vi "灰度分析2.vi"() -> ()   [LabVIEW 2018]
uses:
  <vilib>/vision/NI_Vision_Development_Module.lvlib
panel:
  out "error out":errorcluster
  out "波形图 2":cluster{"x0":sgl, "dx":sgl, "Pixels Line":sgl[]}(graph)
  out "波形图":sgl[](graph)
  out "Image":T1(plugin-control)
  in  "路径":path
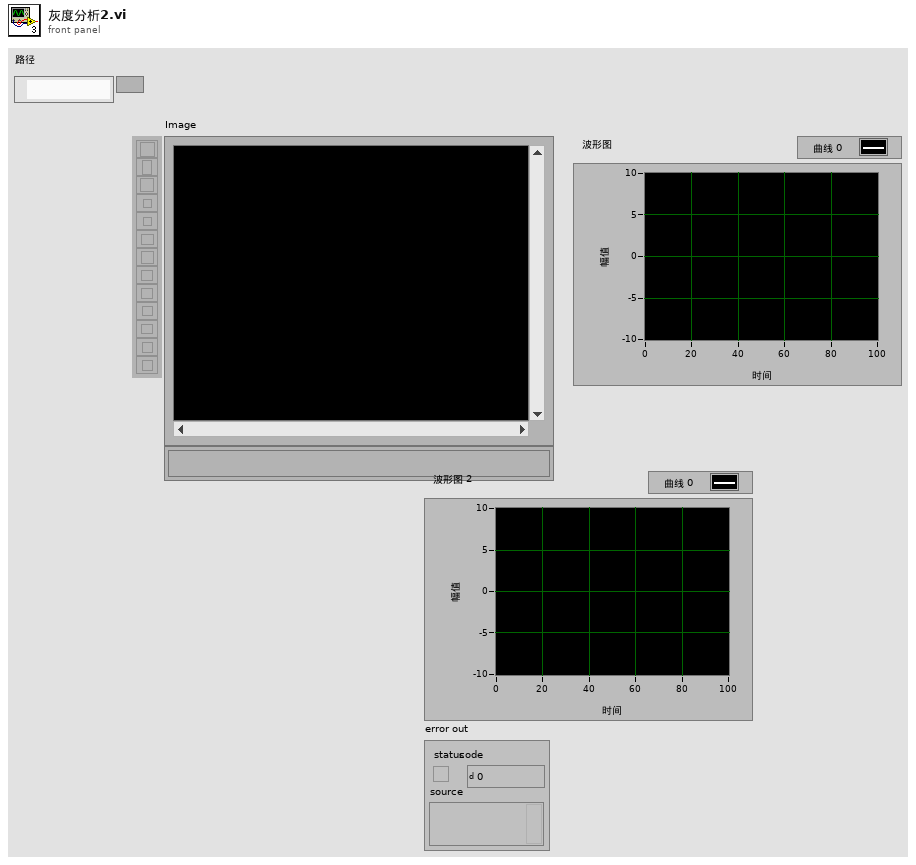
[diagram p1: front panel]
types:
  T1 = typedef "IMAQ Image.ctl" = refnum<image>
  T2 = cluster{"Global Rectangle":i32[], "Contours":cluster{"ID":enum32{"External", "Internal"}, "Type":u32, "Coordinates":i32[]}[]}
  T3 = cluster{"Left":i32, "Top":i32, "Right":i32, "Bottom":i32}
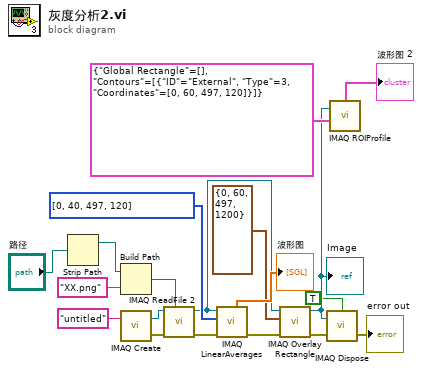
[diagram p0: block diagram]
diagram:
  n1 = Strip Path(path="路径") -> (stripped path=w18:path)  [unwired: 1 out]
  n2 = Build Path(base path=w18, name or relative path="XX.png" ("名称或相对路径")) -> (appended path=w13:path)
  n3 = call "IMAQ Create"("Image Name"="untitled") -> ("New Image"=w16:T1, "error out"=w15:errorcluster)  [unwired: 4 in]
  n4 = call "IMAQ ReadFile 2"("File Path"=w13, "error in (no error)"=w15, "Image"=w16) -> ("error out"=w11:errorcluster, "Image Out"=w9:T1)  [unwired: 4 in, 3 out]
  n5 = call "IMAQ LinearAverages"("error in (no error)"=w11, "Optional Rectangle"=i32[] [0, 40, 497, 120], "Image Src"=w9) -> ("error out"=w8:errorcluster, "X Axis Averages"=→"波形图":sgl[])  [unwired: 4 in, 3 out]
  n6 = call "IMAQ Overlay Rectangle"("error in (no error)"=w8, "Rectangle"=T3 {"Left"=0, "Top"=60, "Right"=497, "Bottom"=1200}, "Image"=w9) -> ("error out"=w7:errorcluster, "Image Out"=w3:T1)  [unwired: 7 in]
  "Image" <- w3
  n7 = call "IMAQ Dispose"("All Images? (No)"=TRUE, "Image"=w3, "error in (no error)"=w7) -> ("error out"=→"error out":errorcluster)  [unwired: 3 in]
  n8 = call "IMAQ ROIProfile"("ROI Descriptor"=T2 {"Global Rectangle"=[], "Contours"=[{"ID"=enum."External", "Type"=3, "Coordinates"=[0, 60, 497, 120]}]}, "Image"=w3) -> ("ROI Graph"=→"波形图 2":cluster{"x0":sgl, "dx":sgl, "Pixels Line":sgl[]})  [unwired: 2 in, 4 out]
